vi "GroupKFold.vi"(6 "Groups":string[][](array[string]), 8 "error in (no error)":errorcluster caption="entrée d'erreur (pas d'erreur)", 9 "y":string[][](array[string]), 10 "X":string[][](array[string]), 11 "GroupKFold":cluster{"n_splits":i32}={"n_splits"=5}) -> (0 "error out":errorcluster caption="sortie d'erreur", 3 "Split":T1(array[cluster]))   [LabVIEW 2020]
doc: "K-fold iterator variant with non-overlapping groups.\n\nThe same group will not appear in two different folds (the number of distinct groups has to be at least equal to the number of folds).\n\nThe folds are approximately balanced in the sense that the number of distinct groups is approximately the same in each fold.\n\nParameters : \n\n- n_splits : int, default=5\nNumber of folds. Must be at least 2.\n\nMethods : Split\n\nParameters : \n\n- X : array-like of shape (n_samples, n_features)\nTraining data, where n_samples is the number of samples and n_features is the number of features.\n\n- y : array-like of shape (n_samples,), default=None\nThe target variable for supervised learning problems.\n\n- groups : array-like of shape (n_samples,)\nGroup labels for the samples used while splitting the dataset into train/test set.\n\nYields : \n\n- train : ndarray\nThe training set indices for that split.\n\n- test : ndarray\nThe testing set indices for that split."
uses:
  GroupKFold.lvclass
panel:
  out "GroupKFold.lvclass":refnum<class "GroupKFold.lvclass">
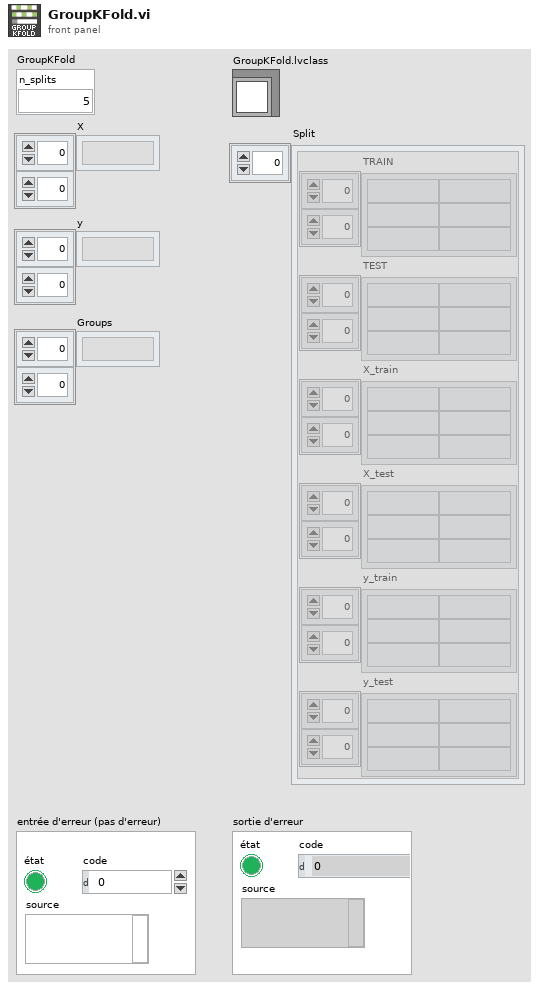
[diagram p1: front panel]
types:
  T1 = cluster{"TRAIN":string[][], "TEST":string[][], "X_train":string[][], "X_test":string[][], "y_train":string[][], "y_test":string[][]}[]
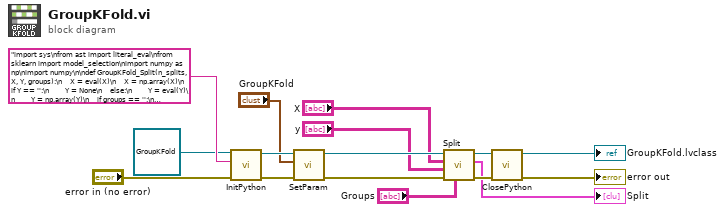
[diagram p0: block diagram]
diagram:
  n1 = call-dynamic "InitPython.vi"("error in (no error)"="error in (no error)", "Python Instruction"="import sys\nfrom ast import literal_eval\nfrom sklearn import model_selection\nimport numpy as np\nimport numpy\n\ndef GroupKFold_Split(n_splits, X, Y, groups):\n    X = eval(X)\n    X = np.array(X)\n    if Y == '':\n        Y = None\n    else:\n        Y = eval(Y)\n        Y = np.array(Y)\n    if groups == '':\n        groups = None\n    else:\n        groups = eval(groups)\n        groups = np.array(groups)\n    list_return = []\n    try:\n        for train_index, test_index in model_selection.GroupKFold(n_splits).split(X, Y, groups):\n            list_return = list_return +[\"TRAIN:\", train_index.tolist(), \"TEST:\", test_index.tolist()]\n            X_train, X_test = X[train_index].tolist(), X[test_index].tolist()\n            y_train, y_test = Y[train_index].tolist(), Y[test_index].tolist()\n            list_return = list_return +[\"X_train:\", X_train, \"X_test:\", X_test, \"y_train:\", y_train, \"y_test:\", y_test]\n        return str(list_return)\n    except:\n        erreur = sys.exc_info()\n        typerr = u\"%s\" % (erreur[0])\n        typerr = typerr[typerr.find(\"'\")+1:typerr.rfind(\"'\")]\n        msgerr = u\"%s\" % (erreur[1])\n        message = str('/!\\\\ {0} : {1}'. format(typerr,msgerr))\n        return message", "Scikit-learn en entrée"=refnum<class "GroupKFold.lvclass"> refnum ("GroupKFold.lvclass")) -> ("error out"=w14:errorcluster, "Scikit-learn en sortie"=w13:refnum<class "GroupKFold.lvclass">)  [unwired: 7 in]
  n2 = call-dynamic "SetParam.vi"("error in (no error)"=w14, "GroupKFold"="GroupKFold", "GroupKFold.lvclass"=w13) -> ("error out"=w9:errorcluster, "GroupKFold.lvclass"=w10:refnum<class "GroupKFold.lvclass">)  [unwired: 7 in]
  n3 = call-dynamic "Split.vi"("Groups"="Groups", "error in (no error)"=w9, "y"="y", "X"="X", "GroupKFold.lvclass"=w10) -> ("error out"=w7:errorcluster, "Split"=→"Split":T1, "GroupKFold.lvclass"=w8:refnum<class "GroupKFold.lvclass">)  [unwired: 4 in]
  n4 = call-dynamic "ClosePython.vi"("error in (no error)"=w7, "Scikit-learn en entrée"=w8) -> ("error out"=→"error out":errorcluster, "Scikit-learn en sortie"=→"GroupKFold.lvclass":refnum<class "GroupKFold.lvclass">)  [unwired: 8 in]
